vi "ConvertMsgParameter.vi"(1 "MSG  Type":enum16{"void", "byte", "int", "float"}(ring), 2 "MSG  PARAM":string) -> (0 "Casted Parameter":i32)   [LabVIEW 2010]
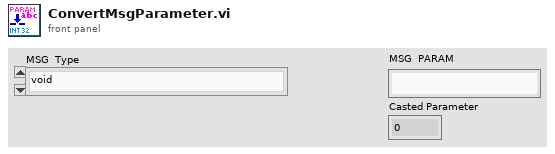
[diagram p1: front panel]
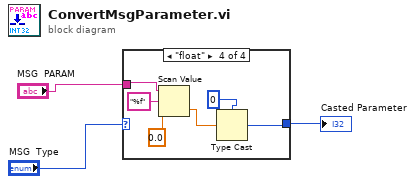
[diagram p0: block diagram]
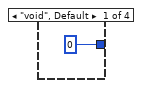
[diagram p2: hidden frame]
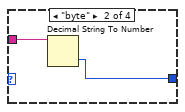
[diagram p3: hidden frame]
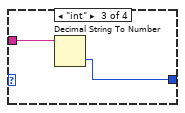
[diagram p4: hidden frame]
diagram:
  n1 = case shown="\"float\"" "MSG  Type" {
    tunnel: "MSG  PARAM" -> [_ w6 w8 w14]
    tunnel: [0 w5 w7 w10] -> w1
    frame "void", Default {
    }
    frame "byte" {
      n2 = Decimal String To Number(string=w6) -> (number=w5:i32)  [unwired: 2 in, 1 out]
    }
    frame "int" {
      n3 = Decimal String To Number(string=w8) -> (number=w7:i32)  [unwired: 2 in, 1 out]
    }
    frame "float" {
      n4 = Scan Value(string=w14, format string="%f", default (0 dbl)=0.0) -> (value=w11:dbl)  [unwired: 1 out]
      n5 = Type Cast(type=0 ("32bit integer"), x=w11) -> (*(type *) &x=w10:i32)
    }
  }
  "Casted Parameter" <- w1
